vi "StateShooter.vi"(1 "Selected State (In)":string) -> (0 "Selected State (Out)":string)   [LabVIEW 2019]
uses:
  dscommands.vi
  outputs.vi
  sensors.vi
  constants.vi
  dsdata.vi
  51c88f72-f87c-413f-8d9c-fe87885b1d16.vi
panel:
  in  "Settling Time (ms)":u32=500
  in  "Max Acceptable Robot Speed (ft/s)":dbl=5.0
  in  "Acceptable Shooter Error Fraction":dbl=0.1
  in  "Shooter Prespin (ms)":u32=7000
  in  "Max Range (in)":dbl=1000.0
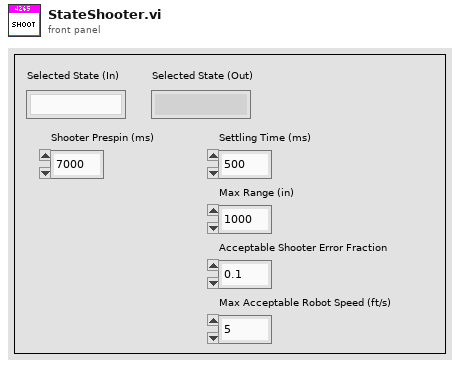
[diagram p1: front panel]
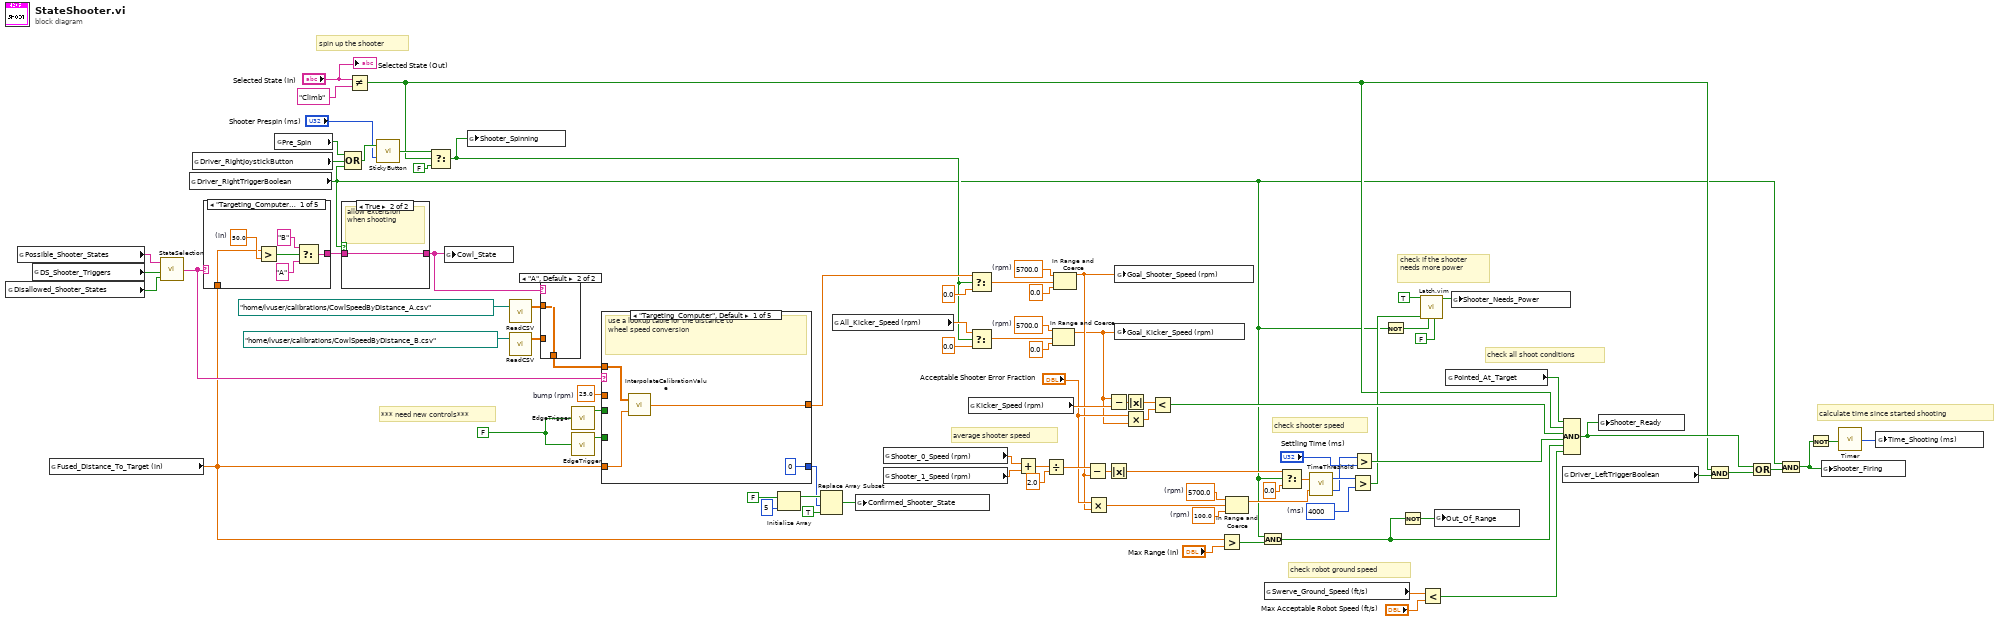
[diagram p0: block diagram]
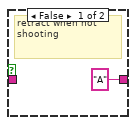
[diagram p2: hidden frame]
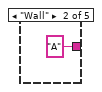
[diagram p3: hidden frame]
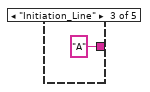
[diagram p4: hidden frame]
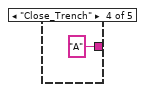
[diagram p5: hidden frame]
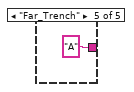
[diagram p6: hidden frame]
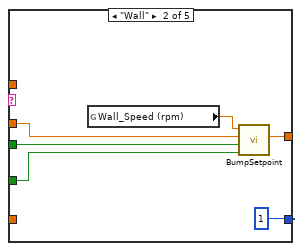
[diagram p8: hidden frame]
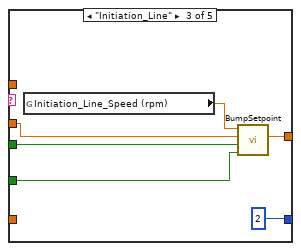
[diagram p9: hidden frame]
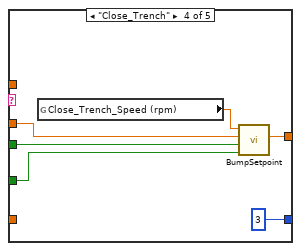
[diagram p10: hidden frame]
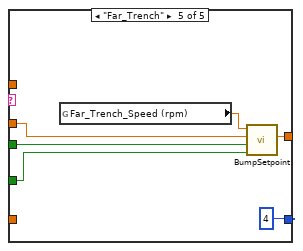
[diagram p11: hidden frame]
diagram:
  w19 = FALSE ("Input Signal")
  w41 = 100.0  # (rpm)
  w42 = 5700.0  # (rpm)
  w50 = 5700.0  # (rpm)
  w22 = 5700.0  # (rpm)
  w53 = u32 4000  # (ms)
  w78 = 25.0  # bump (rpm)
  # "*** need new controls***"
  # "calculate time since started shooting"
  # "check all shoot conditions"
  # "average shooter speed"
  # "check shooter speed"
  # "check robot ground speed"
  # "check if the shooter\nneeds more power"
  # "spin up the shooter"
  n1 = global read "outputs.vi" "Disallowed_Shooter_States"() -> (w77:bool[])
  n2 = global read "constants.vi" "Possible_Shooter_States"() -> (w89:string[])
  n3 = global read "dscommands.vi" "DS_Shooter_Triggers"() -> (w88:bool[])
  n4 = global read "sensors.vi" "Fused_Distance_To_Target (in)"() -> (w69:dbl)
  n5 = call "StateSelection.vi"("Disallowed States"=w77, "State Triggers"=w88, "State Names"=w89) -> ("Selected State"=w70:string)
  n6 = global read "dscommands.vi" "Driver_RightTriggerBoolean"() -> (w2:bool)
  n7 = global read "dscommands.vi" "Driver_RightJoystickButton"() -> (w66:bool)
  n8 = case shown="\"Targeting_Computer\", Default" w70 {
    tunnel: [w90 "A" ("A,B,C") "A" ("A,B,C") "A" ("A,B,C") "A" ("A,B,C")] -> w71
    tunnel: w69 -> [w91 _ _ _ _]
    frame "Targeting_Computer", Default {
      w92 = 50.0  # (in)
      n9 = Greater?(x=w91, y=w92) -> (0:w95:bool)
      n10 = Select(t="B", s=w95, f="A") -> (s? t:f=w90:string)
    }
    frame "Wall" {
    }
    frame "Initiation_Line" {
    }
    frame "Close_Trench" {
    }
    frame "Far_Trench" {
    }
  }
  n11 = global read "dscommands.vi" "Pre_Spin"() -> (w20:bool)
  n12 = case shown="True" w2 {
    tunnel: w71 -> [_ w101]
    tunnel: ["A" ("A,B,C") w101] -> w17
    frame False {
      # "retract when not shooting"
    }
    frame True {
      # "allow extension when shooting"
    }
  }
  n13 = Compound Arithmetic op=OR(w20, w66, w2) -> (w65:bool)
  n14 = Not Equal?(x="Selected State (In)", y="Climb") -> (x != y?=w3:bool)
  n15 = call "StickyButton.vi"("Time threshold (ms)"="Shooter Prespin (ms)", "Button Input"=w65) -> ("Sticky Button"=w10:bool)
  n16 = Select(t=w10, s=w3, f=FALSE ("t")) -> (s? t:f=w18:bool)
  n17 = global write "outputs.vi" "Cowl_State"(w17) -> ()
  n18 = global write "outputs.vi" "Shooter_Spinning"(w18) -> ()
  n19 = call "ReadCSV.vi"("File Path (.csv)"=path "/home/lvuser/calibrations/CowlSpeedByDistance_A.csv" ("path")) -> ("Data (index by row)"=w74:dbl[][])  [unwired: 1 in, 1 out]
  n20 = call "ReadCSV.vi"("File Path (.csv)"=path "/home/lvuser/calibrations/CowlSpeedByDistance_B.csv" ("path")) -> ("Data (index by row)"=w73:dbl[][])  [unwired: 1 in, 1 out]
  n21 = case shown="\"A\", Default" w17 {
    tunnel: w74 -> [_ w103]
    tunnel: w73 -> [w102 _]
    tunnel: [w102 w103] -> w72
    frame "B" {
    }
    frame "A", Default {
    }
  }
  n22 = call "EdgeTrigger.vi"("Input Signal"=w19) -> ("Rising Edge Trigger"=w80:bool)  [unwired: 2 out]
  n23 = call "EdgeTrigger.vi"("Input Signal"=w19) -> ("Rising Edge Trigger"=w79:bool)  [unwired: 2 out]
  n24 = case shown="\"Targeting_Computer\", Default" w70 {
    tunnel: [0 1 2 3 4] -> w82
    tunnel: w69 -> [w106 _ _ _ _]
    tunnel: w80 -> [_ w110 w117 w121 w127]
    tunnel: w79 -> [_ w109 w116 w122 w128]
    tunnel: w78 -> [_ w111 w114 w120 w126]
    tunnel: w72 -> [w104 _ _ _ _]
    tunnel: [w105 w108 w115 w123 w129] -> w30
    frame "Targeting_Computer", Default {
      # "use a lookup table for the distance to\nwheel speed conversion"
      n25 = call "InterpolateCalibrationValue.vi"("Input"=w106, "Calibration Data"=w104) -> ("Interpolated Output"=w105:dbl)
    }
    frame "Wall" {
      n26 = global read "dsdata.vi" "Wall_Speed (rpm)"() -> (w112:dbl)
      n27 = call "BumpSetpoint.vi"("Bump Down Trigger"=w109, "Bump Up Trigger"=w110, "Bump Increment"=w111, "Original Setpoint"=w112) -> ("Bumped Setpoint"=w108:dbl)  [unwired: 7 in]
    }
    frame "Initiation_Line" {
      n28 = global read "dsdata.vi" "Initiation_Line_Speed (rpm)"() -> (w118:dbl)
      n29 = call "BumpSetpoint.vi"("Bump Down Trigger"=w116, "Bump Up Trigger"=w117, "Bump Increment"=w114, "Original Setpoint"=w118) -> ("Bumped Setpoint"=w115:dbl)  [unwired: 7 in]
    }
    frame "Close_Trench" {
      n30 = global read "dsdata.vi" "Close_Trench_Speed (rpm)"() -> (w124:dbl)
      n31 = call "BumpSetpoint.vi"("Bump Down Trigger"=w122, "Bump Up Trigger"=w121, "Bump Increment"=w120, "Original Setpoint"=w124) -> ("Bumped Setpoint"=w123:dbl)  [unwired: 7 in]
    }
    frame "Far_Trench" {
      n32 = global read "dsdata.vi" "Far_Trench_Speed (rpm)"() -> (w130:dbl)
      n33 = call "BumpSetpoint.vi"("Bump Down Trigger"=w128, "Bump Up Trigger"=w127, "Bump Increment"=w126, "Original Setpoint"=w130) -> ("Bumped Setpoint"=w129:dbl)  [unwired: 7 in]
    }
  }
  n34 = Initialize Array(FALSE, 5 ("dimension size")) -> (w85:bool[])
  n35 = Replace Array Subset(array=w85, new element=TRUE ("new element/subarray"), index=w82) -> (w83:bool[])
  n36 = global read "dsdata.vi" "All_Kicker_Speed (rpm)"() -> (w48:dbl)
  n37 = global write "outputs.vi" "Confirmed_Shooter_State"(w83) -> ()
  n38 = global read "sensors.vi" "Shooter_0_Speed (rpm)"() -> (w61:dbl)
  n39 = global read "sensors.vi" "Shooter_1_Speed (rpm)"() -> (w60:dbl)
  n40 = global read "sensors.vi" "Kicker_Speed (rpm)"() -> (w46:dbl)
  n41 = Select(t=w30, s=w18, f=0.0) -> (s? t:f=w52:dbl)
  n42 = Select(t=w48, s=w18, f=0.0) -> (s? t:f=w47:dbl)
  n43 = Add(x=w61, y=w60) -> (x+y=w59:dbl)
  n44 = Divide(x=w59, y=2.0) -> (x/y=w56:dbl)
  n45 = In Range and Coerce(upper limit=w50, x=w47, lower limit=0.0) -> (coerced(x)=w31:dbl)  [unwired: 1 out]
  n46 = In Range and Coerce(upper limit=w22, x=w52, lower limit=0.0) -> (coerced(x)=w37:dbl)  [unwired: 1 out]
  n47 = Subtract(x=w56, y=w37) -> (x-y=w57:dbl)
  n48 = Multiply(x="Acceptable Shooter Error Fraction", y=w37) -> (x*y=w40:dbl)
  n49 = Subtract(x=w31, y=w46) -> (x-y=w45:dbl)
  n50 = Absolute Value(x=w57) -> (abs(x)=w36:dbl)
  n51 = global write "outputs.vi" "Goal_Shooter_Speed (rpm)"(w37) -> ()
  n52 = global write "outputs.vi" "Goal_Kicker_Speed (rpm)"(w31) -> ()
  n53 = Absolute Value(x=w45) -> (abs(x)=w38:dbl)
  n54 = Multiply(x="Acceptable Shooter Error Fraction", y=w31) -> (x*y=w43:dbl)
  n55 = Less?(x=w38, y=w43) -> (x < y?=w21:bool)
  n56 = Greater?(x=w69, y="Max Range (in)") -> (0:w29:bool)
  n57 = In Range and Coerce(upper limit=w42, x=w40, lower limit=w41) -> (coerced(x)=w39:dbl)  [unwired: 1 out]
  n58 = And(x=w2, y=w29) -> (x .and. y?=w1:bool)
  n59 = global read "sensors.vi" "Swerve_Ground_Speed (ft/s)"() -> (w16:dbl)
  n60 = Select(t=w36, s=w2, f=0.0) -> (s? t:f=w35:dbl)
  n61 = call "TimeThreshold.vi"("Threshold"=w39, "Current Value"=w35) -> ("Time Below Threshold (ms)"=w33:u32, "Time Above Threshold (ms)"=w54:u32)
  n62 = Greater?(x=w54, y=w53) -> (0:w14:bool)
  n63 = Greater?(x=w33, y="Settling Time (ms)") -> (0:w24:bool)
  n64 = Not(x=w2) -> (.not. x?=w12:bool)
  n65 = Not(x=w1) -> (.not. x?=w8:bool)
  n66 = call "Latch.vim"("Default Value"=FALSE, "Reset"=w12, "Latch Signal"=w14, "Latch Value"=TRUE) -> ("Latched"=w11:bool)  [unwired: 7 in]
  n67 = Less?(x=w16, y="Max Acceptable Robot Speed (ft/s)") -> (x < y?=w23:bool)
  n68 = global write "outputs.vi" "Out_Of_Range"(w8) -> ()
  n69 = global read "sensors.vi" "Pointed_At_Target"() -> (w7:bool)
  n70 = global write "outputs.vi" "Shooter_Needs_Power"(w11) -> ()
  n71 = global read "dscommands.vi" "Driver_LeftTriggerBoolean"() -> (w28:bool)
  n72 = Compound Arithmetic op=AND(w7, w3, w21, w24, w1, w23) -> (w6:bool)
  n73 = global write "outputs.vi" "Shooter_Ready"(w6) -> ()
  n74 = Compound Arithmetic op=AND(w3, w28) -> (w27:bool)
  n75 = Compound Arithmetic op=OR(w6, w27) -> (w5:bool)
  n76 = Compound Arithmetic op=AND(w2, w5) -> (w4:bool)
  n77 = Not(x=w4) -> (.not. x?=w26:bool)
  n78 = global write "outputs.vi" "Shooter_Firing"(w4) -> ()
  n79 = call "Timer.vi"("Reset Timer"=w26) -> ("Time (ms)"=w25:u32)
  n80 = global write "outputs.vi" "Time_Shooting (ms)"(w25) -> ()
  "Selected State (Out)" <- "Selected State (In)"
